vi "Stop Condition.vi"(11 "Light Sensor Array":i32[](array[numeric])) -> (3 "element":bool)   [LabVIEW 2018]
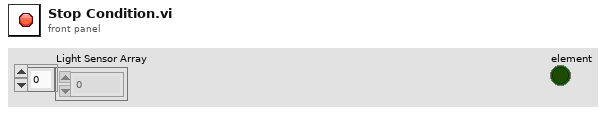
[diagram p1: front panel]
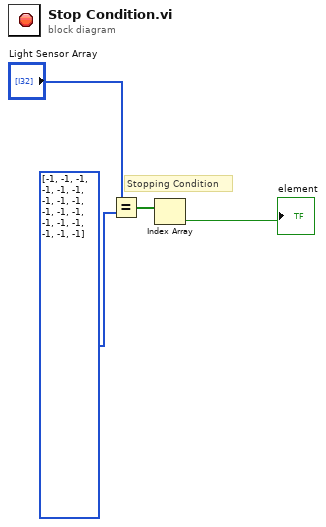
[diagram p0: block diagram]
diagram:
  # "Stopping Condition"
  n1 = Equal?(x="Light Sensor Array", y=i32[] [-1, -1, -1, -1, -1, -1, -1, -1, -1, -1, -1, -1, -1, -1, -1, -1, -1, -1] ("Array")) -> (x = y?=w3:bool[])
  n2 = Index Array(array=w3) -> (element=→"element":bool)  [unwired: 1 in]
